vi "Set Calibration.vi"() -> ()   [LabVIEW 2018, in "Configuration.lvlib"]
uses:
  Configuration.lvlib
  Configuration.lvclass
panel:
  out "Calibration Data:":string
  in  "Calibration Required?":bool
  in  "Device":string="Optical Power Meter"
  in  "Select Device":bool
  in  "New Calibration Date":timestamp
  in  "Update Cal":bool
  in  "Read Cal":bool
  in  "stop":bool
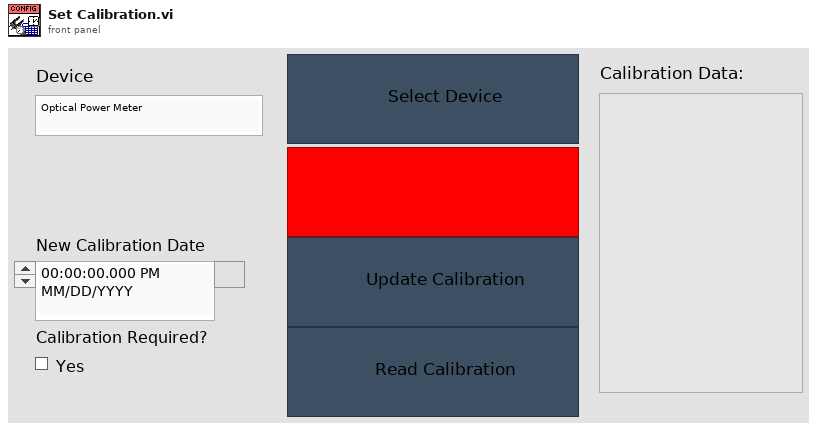
[diagram p1: front panel]
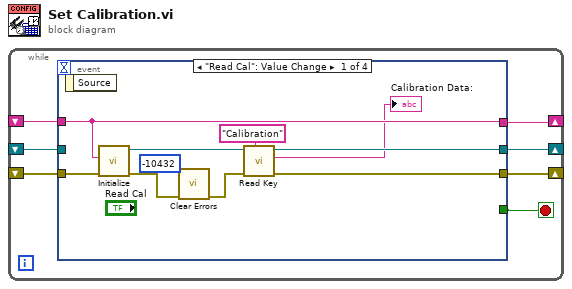
[diagram p0: block diagram]
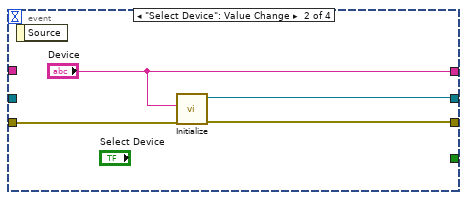
[diagram p2: hidden frame]
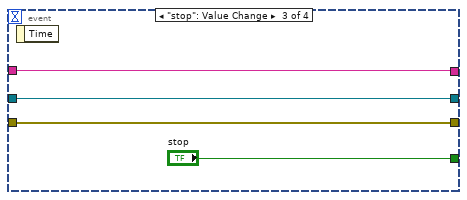
[diagram p3: hidden frame]
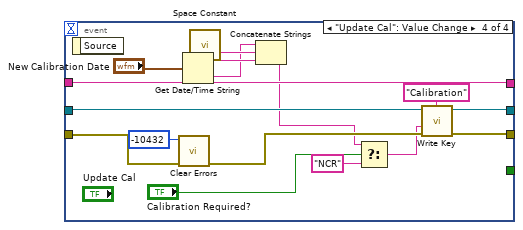
[diagram p4: hidden frame]
diagram:
  n1 = while {
    shift-right: [w5] -> _
    shift-left: _ -> [w6]
    shift-right: [w3] -> _
    shift-left: _ -> [w4]
    shift-right: [w1] -> _
    shift-left: _ -> [w2]
    stop <- w7 stop-if-true
    n2 = event shown="[0] \"Read Cal\": Value Change" {
      selector: _ -> [_ _ _ _]
      dyn-events: _ -> [_ _ _ _]
      timeout: _ -> [_ _ _ _]
      tunnel: [_ _ "stop" _] -> w7
      tunnel: w6 -> [w14 w21 w24 w33]
      tunnel: [w16 w20 w24 w41] -> w5
      tunnel: w4 -> [_ _ w23 w39]
      tunnel: [w17 w19 w23 w40] -> w3
      tunnel: w2 -> [w12 _ w22 w34]
      tunnel: [w12 "Device" w22 w34] -> w1
      event "Read Cal": Value Change {
        n3 = event-data() -> ()  [unwired: 1 in, 1 out]
        n4 = call "Initialize.vi"("error in"=w14, "Device"=w12) -> ("error out"=w13:errorcluster, "Configuration out"=w11:refnum<class "Configuration.lvclass">)  [unwired: 8 in]
        n5 = call <vilib>:"Clear Errors.vi"("error in (no error)"=w13, "specific error code to clear (0: all)"=-10432) -> ("error out"=w10:errorcluster)  [unwired: 4 in, 1 out]
        n6 = call "Read Key.vi"("Key:"="Calibration", "error in"=w10, "Configuration in"=w11) -> ("error out"=w16:errorcluster, "Value"=→"Calibration Data:":string, "Configuration out"=w17:refnum<class "Configuration.lvclass">)  [unwired: 6 in]
      }
      event "Select Device": Value Change {
        n7 = event-data() -> ()  [unwired: 1 in, 1 out]
        n8 = call "Initialize.vi"("error in"=w21, "Device"="Device") -> ("error out"=w20:errorcluster, "Configuration out"=w19:refnum<class "Configuration.lvclass">)  [unwired: 8 in]
      }
      event "stop": Value Change {
        n9 = event-data() -> ()  [unwired: 1 in, 1 out]
      }
      event "Update Cal": Value Change {
        n10 = event-data() -> ()  [unwired: 1 in, 1 out]
        n11 = call <vilib>:"Clear Errors.vi"("error in (no error)"=w33, "specific error code to clear (0: all)"=-10432) -> ("error out"=w32:errorcluster)  [unwired: 4 in, 1 out]
        n12 = Get Date/Time String(seconds (now)="New Calibration Date") -> (date string=w37:string, time string=w35:string)  [unwired: 2 in]
        n13 = call <vilib>:"Space Constant.vi"() -> ("String"=w36:string)
        n14 = Concatenate Strings(w35, w36, w37) -> (w29:string)
        n15 = Select(t=w29, s="Calibration Required?", f="NCR") -> (s? t:f=w28:string)
        n16 = call "Write Key.vi"("error in"=w32, "value"=w28, "key"="Calibration", "Configuration in"=w39) -> ("error out"=w41:errorcluster, "Configuration out"=w40:refnum<class "Configuration.lvclass">)  [unwired: 6 in]
      }
    }
  }
